vi "PH_Beckhoff_PP_PU.evt Call Reconfigure.vi"(0 "i ref in":refnum<vi>, 2 "Instance name":T1, 5 "error in":errorcluster) -> (14 "i ref out":refnum<vi>, 19 "error out":errorcluster)   [LabVIEW 2014, in "PH_Beckhoff_PP_PU.lvlib"]
doc: "This VI calls an event by a simple call."
uses:
  PH_Beckhoff_PP_PU.lvlib
  PH_Basics/PH_PP_Common/PH_PP_Common.PUs.ctl
  CS_Core/BaseProcess/BaseProcess.lvlib
  PH_Basics/PH_PP_Common/PH_PP_Common.lvlib
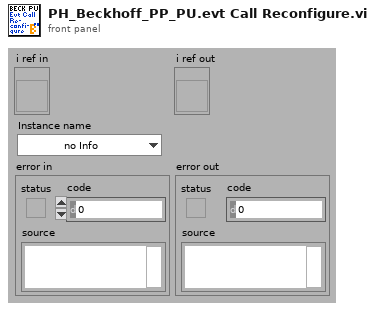
[diagram p1: front panel]
types:
  T1 = typedef "PH_PP_Common.lvlib/PH_PP_Common.PUs.ctl" = enum16{"no Info", "PA-19mm-1", "PA-19mm-2", "PA-45mm-PILC", "PA-45mm-MAIN", "MA-PU-1", "MA-PU-2", "MA-PU-3", "MA-PU-4", "MA-PU-5", "MA-PU-6", "MA-FR", "MA-PILC", "PA-45mm-DP"}
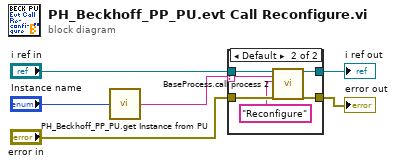
[diagram p0: block diagram]
diagram:
  n1 = call "PH_Beckhoff_PP_PU.get Instance from PU.vi"("PU"="Instance name") -> ("Beckhoff PU Instance"=w1:string)
  n2 = case shown="Default" w1 {
    selector: w1 -> [_ w10]
    tunnel: [w7 w12] -> w6
    tunnel: "error in" -> [w7 w11]
    tunnel: [w8 w13] -> w4
    tunnel: "i ref in" -> [w8 w14]
    frame "", "N/A" {
    }
    frame Default {
      n3 = call "BaseProcess.call process 2.vi"("i ref in"=w14, "Object"=w10, "Selector"="Reconfigure", "error in (no error)"=w11) -> ("i ref out"=w13:refnum<vi>, "error out"=w12:errorcluster)  [unwired: 14 in]
    }
  }
  "error out" <- w6
  "i ref out" <- w4
